vi "Configure Subsequent Measurement.vi"(8 "error in (no error)":errorcluster, 10 "Measurement Function (0: Current)":i32(ring) items=["Current", "Resistance", "Charge"], 11 "VISA resource name":refnum<visa-resource-name>) -> (0 "error out":errorcluster, 3 "VISA resource name out":refnum<visa-resource-name>)   [LabVIEW 2019, in "Keithley 6517.lvlib"]
doc: "Configures the instrument for subsequent measurements on the specified function (Current, Resistance, and Charge). Basically, it places the instrument in a one-shot measurement mode.\n\nNote:\nPlease configure the specified function first by <b>Configure Measurement Function.vi.</b>"
uses:
  Keithley 6517.lvlib
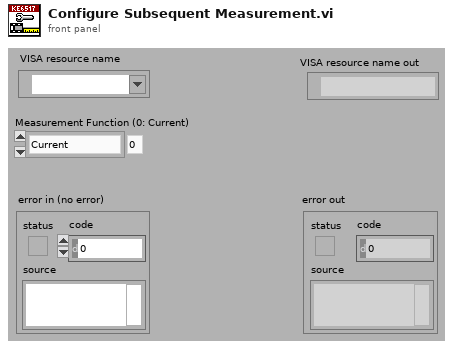
[diagram p1: front panel]
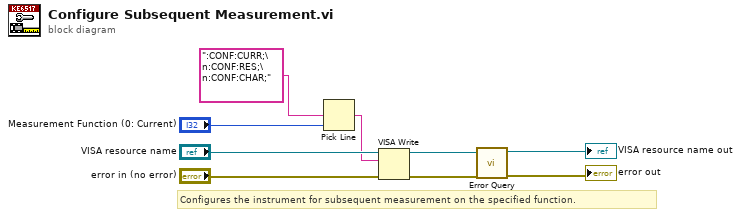
[diagram p0: block diagram]
diagram:
  # "Configures the instrument for subsequent measurement on the specified function."
  n1 = Pick Line(multi-line string=":CONF:CURR;\n:CONF:RES;\n:CONF:CHAR;", line index="Measurement Function (0: Current)") -> (output string=w1:string)  [unwired: 1 in]
  n2 = VISA Write(VISA resource name="VISA resource name", write buffer=w1, error in (no error)="error in (no error)") -> (VISA resource name out=w7:refnum<visa-resource-name>, error out=w6:errorcluster)  [unwired: 1 out]
  n3 = call "Error Query.vi"("error in (no error)"=w6, "VISA resource name"=w7) -> ("error out"=→"error out":errorcluster, "VISA resource name out"=→"VISA resource name out":refnum<visa-resource-name>)  [unwired: 6 in, 2 out]
